vi "Log Warnings.vi"(8 "Error In":errorcluster, 10 "Weather Data":T1, 11 "file ref in":refnum<file>) -> (0 "Error Out":errorcluster, 3 "file ref out":refnum<file>)   [LabVIEW 2019]
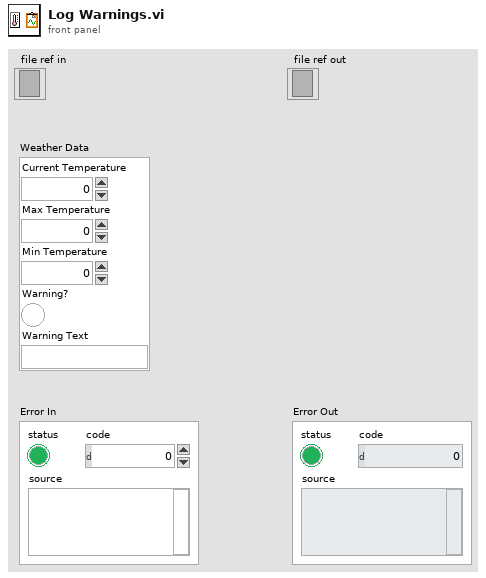
[diagram p1: front panel]
types:
  T1 = cluster{"Current Temperature":dbl, "Max Temperature":dbl, "Min Temperature":dbl, "Warning?":bool, "Warning Text":string}
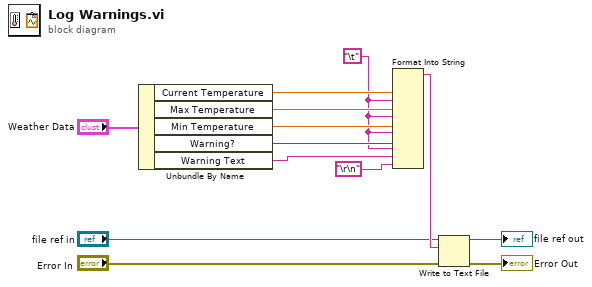
[diagram p0: block diagram]
diagram:
  w7 = "\t"
  n1 = Unbundle By Name("Weather Data") -> ("Current Temperature"=w12:dbl, "Max Temperature"=w11:dbl, "Min Temperature"=w10:dbl, "Warning?"=w9:bool, "Warning Text"=w8:string)
  n2 = Format Into String(w12, w7, w11, w7, w10, w7, w9, w7, w8, "\r\n") -> (resulting string=w5:string)  [unwired: 3 in, 1 out]
  n3 = Write to Text File(file (use dialog)="file ref in", text=w5, error in="Error In") -> (refnum out=→"file ref out":refnum<file>, error out=→"Error Out":errorcluster)  [unwired: 1 in, 1 out]
